vi "test.vi"() -> ()   [LabVIEW 2015]
uses:
  <vilib>/NXT/Block Support/NXT_InputPort.ctl
  <vilib>/NXT/Block Support/NXT_OutputPort.ctl
  <vilib>/NXT/Dual Mode Library/Sensors/Light_On.vi
  <vilib>/NXT/NXTIO Xnodes/NXTIONodeSubVIs/NXTMoveMotors.vi
  <vilib>/NXT/NXTIO Xnodes/NXTIONodeSubVIs/NXTStopMotors.vi
  <vilib>/NXT/NXTIO Xnodes/AddressXNode/NXTIOAddress.xnode
  <vilib>/NXT/Subs/LVHSConnector.ctl
  <vilib>/NXT/NXTIO Xnodes/NXTIOXNode/NXTIO.xnode
  <vilib>/NXT/LegoClasses/BrickReference/BrickReference.lvclass
panel:
  in  "stop":bool
  in  "Power/Speed 1":i8=75
  in  "오른쪽 port1":T1=2 items=["Port 1", "Port 2", "Port 3", "Port 4"]
  in  "왼쪽 port4":T1=2 items=["Port 1", "Port 2", "Port 3", "Port 4"]
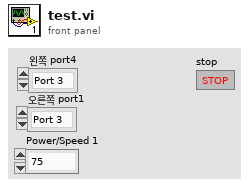
[diagram p1: front panel]
types:
  T1 = typedef "NXT_InputPort.ctl" = u32
  T2 = typedef "NXT_OutputPort.ctl" = u8
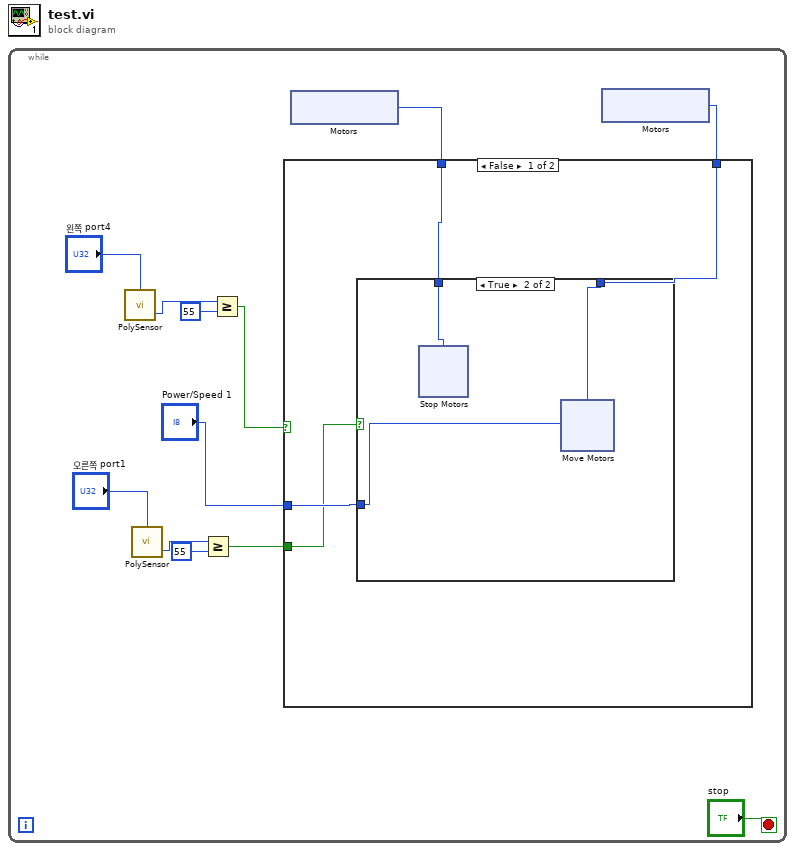
[diagram p0: block diagram]
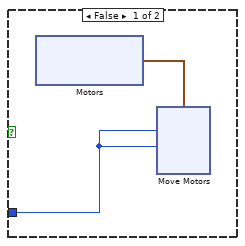
[diagram p2: hidden frame]
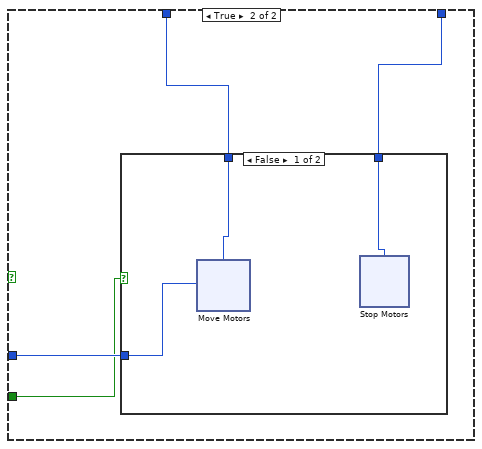
[diagram p3: hidden frame]
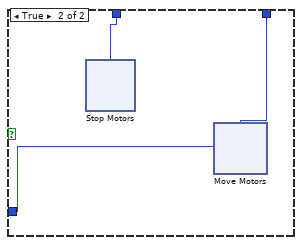
[diagram p4: hidden frame]
diagram:
  n1 = while {
    stop <- "stop" stop-if-true
    n2 = call-poly <vilib>:"PolySensor.vi"("Port (Port 3)"="왼쪽 port4") -> ("Scaled Value"=w8:i16)  [unwired: 2 in, 1 out]
    n3 = call-poly <vilib>:"PolySensor.vi"("Port (Port 3)"="오른쪽 port1") -> ("Scaled Value"=w9:i16)  [unwired: 2 in, 1 out]
    n4 = Greater Or Equal?(x=w9, y=i16 55) -> (x >= y?=w5:bool)
    n5 = Greater Or Equal?(x=w8, y=i16 55) -> (x >= y?=w4:bool)
    n6 = xnode "Motors"() -> ("Motor"=w2:T2)
    n7 = xnode "Motors"() -> ("Motor"=w1:T2)
    n8 = case shown="False" w4 {
      tunnel: "Power/Speed 1" -> [w18 w48]
      tunnel: w5 -> [w17 w45]
      tunnel: w2 -> [w16 w47]
      tunnel: w1 -> [w15 w46]
      frame False {
        n9 = case shown="True" w17 {
          tunnel: w18 -> [w19 w31]
          tunnel: w16 -> [_ w30]
          tunnel: w15 -> [_ w32]
          frame False {
            n10 = xnode "Motors"() -> ("Motor"=w20:cluster{"Port":T2, "Port":T2})
            n11 = xnode "Move Motors"("Power/Speed 2"=w19, "Power/Speed 1"=w19, "Motors"=w20) -> ()  [unwired: 1 in, 1 out]
          }
          frame True {
            n12 = xnode "Stop Motors"("Motors"=w30) -> ()  [unwired: 1 in, 1 out]
            n13 = xnode "Move Motors"("Power/Speed 1"=w31, "Motors"=w32) -> ()  [unwired: 1 in, 1 out]
          }
        }
      }
      frame True {
        n14 = case shown="False" w45 {
          tunnel: w48 -> [w49 w65]
          tunnel: w47 -> [w50 w64]
          tunnel: w46 -> [w51 w66]
          frame False {
            n15 = xnode "Move Motors"("Power/Speed 1"=w49, "Motors"=w50) -> ()  [unwired: 1 in, 1 out]
            n16 = xnode "Stop Motors"("Motors"=w51) -> ()  [unwired: 1 in, 1 out]
          }
          frame True {
            n17 = xnode "Stop Motors"("Motors"=w64) -> ()  [unwired: 1 in, 1 out]
            n18 = xnode "Move Motors"("Power/Speed 1"=w65, "Motors"=w66) -> ()  [unwired: 1 in, 1 out]
          }
        }
      }
    }
  }
